vi "PC_Host_LED_Controller.vi"() -> ()   [LabVIEW 2019]
panel:
  in  "stop":bool
  in  "Commande LED":bool
  out "Valeur capteur":dbl
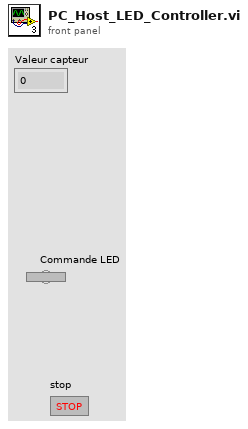
[diagram p1: front panel]
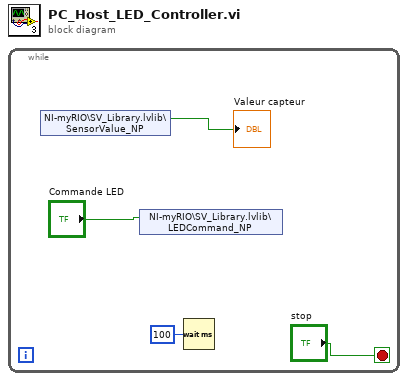
[diagram p0: block diagram]
diagram:
  n1 = while {
    stop <- "stop" stop-if-true
    n2 = shared-variable "NI-myRIO\\SV_Library.lvlib\\SensorValue_NP"() -> (→"Valeur capteur":bool)  [unwired: 1 in, 1 out]
    n3 = shared-variable "NI-myRIO\\SV_Library.lvlib\\LEDCommand_NP"("Commande LED") -> ()  [unwired: 1 in, 1 out]
    n4 = Wait (ms)(milliseconds to wait=u32 100) -> ()  [unwired: 1 out]
  }
